vi "Find Wire To-From.vi"(9 "Wires":T1[](array[typedef]), 10 "termUUID":string, 11 "From UUID?":bool) -> (1 "Found":bool, 2 "Index":i32, 3 "Wire":T1)   [LabVIEW 2025]
uses:
  Controls/wire.ctl
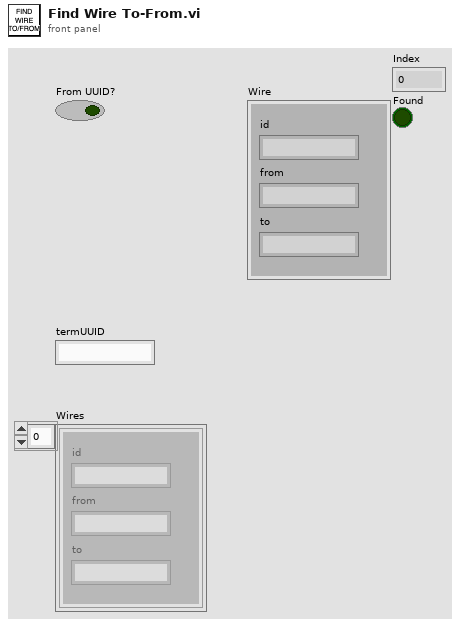
[diagram p1: front panel]
types:
  T1 = typedef "wire.ctl" = cluster{"id":string, "from":string, "to":string}
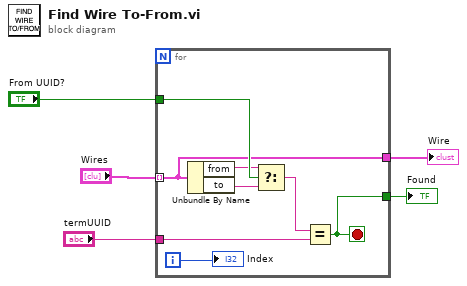
[diagram p0: block diagram]
diagram:
  n1 = for {
    tunnel: "Wires" -> [w8] mode=indexing
    tunnel: "From UUID?" -> [w13]
    tunnel: "termUUID" -> [w9]
    tunnel: [w8] -> w5
    tunnel: [w6] -> w1
    i -> [w7]
    stop <- w6 stop-if-true
    n2 = Unbundle By Name(w8) -> ("from"=w11:string, "to"=w12:string)
    n3 = Select(t=w11, s=w13, f=w12) -> (s? t:f=w10:string)
    n4 = Equal?(x=w10, y=w9) -> (x = y?=w6:bool)
    "Index" <- w7
  }
  "Wire" <- w5
  "Found" <- w1
